vi "Control_Interface_v1.8_cfg.vi"() -> ()   [LabVIEW 2019]
uses:
  Users/zhuen/AppData/Local/CETONI_SDK/lib/labview/labbCAN_Bus_API/labbCAN_Bus_API.lvlib
  Users/zhuen/AppData/Local/CETONI_SDK/lib/labview/labbCAN_Pump_API/labbCAN_Pump_API.lvlib
  Users/zhuen/AppData/Local/CETONI_SDK/lib/labview/labbCAN_Bus_API/TimeUnits.ctl
  Users/zhuen/AppData/Local/CETONI_SDK/lib/labview/labbCAN_Pump_API/VolumeUnits.ctl
  Users/zhuen/AppData/Local/CETONI_SDK/lib/labview/labbCAN_Bus_API/SiUnitPrefix.ctl
panel:
  in  "Tab Control":enum32{"Tracker", "Pump"}(tab)
  in  "Automation":enum16{"OFF", "ON"}(ring)
  in  "Bit Size":enum16{"Auto", "8 bit", "12 bit", "16 bit"}(ring)
  out "Error out Python":errorcluster
  in  "Capture Mode":T1(ring)
  in  "Start Tracker":bool
  out "Tracker  Working":bool
  in  "Browse Capture Path":path
  in  "Capture Path":bool
  in  "File Name":string
  out "Communication Board":string
  in  "Microscopy":enum16{"Fluorescence", "Bright Field"}(ring)
  in  "Tracking Method":enum16{"Contour", "Motion"}(ring)
  in  "Connect":bool
  out "Connected":bool
  out "Config Path":string
  out "Syringe":dbl(slide) caption="Syringe level (ml)" min=0.0 max=10.0 scale=0.0..10.0 scale format="%.1g"
  out "pumping":bool
  in  "SetSyringeLevel":bool
  in  "Generate Flow":bool
  in  "Refill":bool
  in  "Empty":bool
  in  "Stop Dosage":bool
  out "Actual flow rate":dbl caption="Flow rate (ul/min)" format="%#.2g"
  in  "Target Syr Level":dbl caption="Syringe level (ml)" min=0.0 max=10.0 step=1.0 format="%.2g"
  in  "Flow rate":dbl caption="Flow rate (ul/min)" min=-62103.597908503194 max=62103.597908503194 step=1.0 format="%.2g"
  out "Syringe 2":dbl(slide) caption="Syringe level (ml)" min=0.0 max=10.0 scale=0.0..10.0 scale format="%.1g"
  in  "Target Syr Level 2":dbl caption="Syringe level (ml)" min=0.0 max=10.0 step=1.0 format="%.2g"
  in  "Flow rate 2":dbl caption="Flow rate (ul/min)" min=-67160.37941759253 max=67160.37941759253 step=1.0 format="%.2g"
  in  "Stop Dosage 2":bool
  in  "Refill 2":bool
  out "Actual flow rate 2":dbl caption="Flow rate (ul/min)" format="%#.2g"
  out "pumping 2":bool
  in  "Empty 2":bool
  in  "Generate Flow 2":bool
  in  "SetSyringeLevel 2":bool
  out "Syringe 3":dbl(slide) caption="Syringe level (ml)" min=0.0 max=10.0 scale=0.0..10.0 scale format="%.1g"
  in  "Target Syr Level 3":dbl caption="Syringe level (ml)" min=0.0 max=10.0 step=1.0 format="%.2g"
  in  "Flow rate 3":dbl caption="Flow rate (ul/min)" min=-70023.0288619775 max=70023.0288619775 step=1.0 format="%.2g"
  in  "Stop Dosage 3":bool
  in  "Refill 3":bool
  out "Actual flow rate 3":dbl caption="Flow rate (ul/min)" format="%#.2g"
  out "pumping 3":bool
  in  "Empty 3":bool
  in  "Generate Flow 3":bool
  in  "SetSyringeLevel 3":bool
  in  "Total Flow Rate":sgl caption="Total Flow Rate (ul/min)" min=0 max=62103.6 step=1 format="%.2g"
  in  "Stop Dosage All":bool
  in  "Generate Flow All":bool
  out "error out":errorcluster caption="Error pump 1"
  out "error out 2":errorcluster caption="Error pump 2"
  out "error out 3":errorcluster caption="Error pump 3"
  out "Pump handle 3":i64
  out "Pump handle 2":i64
  out "Pump handle":i64
  in  "Interrupt":bool
  in  "Exit":bool
  # "Commands"
  # "Pump"
  # "Target"
  # "Target"
  # "Target"
  # "Actual"
  # "Actual"
  # "Actual"
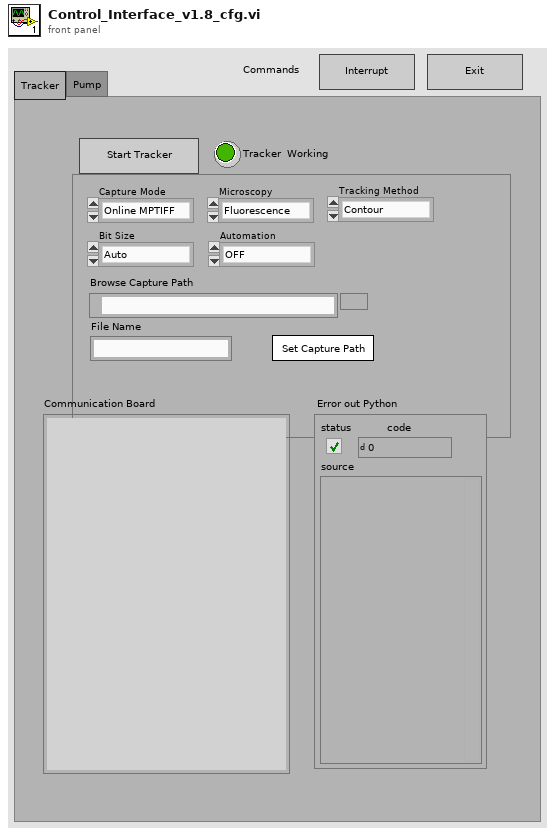
[diagram p1: front panel]
types:
  T1 = enum16{"Online MPTIFF", "Online TIFF", "Offline TIFF"}
  T2 = typedef "labbCAN_Bus_API.lvlib/TimeUnits.ctl" = i32
  T3 = typedef "labbCAN_Pump_API.lvlib/VolumeUnits.ctl" = i32
  T4 = typedef "labbCAN_Bus_API.lvlib/SiUnitPrefix.ctl" = i32
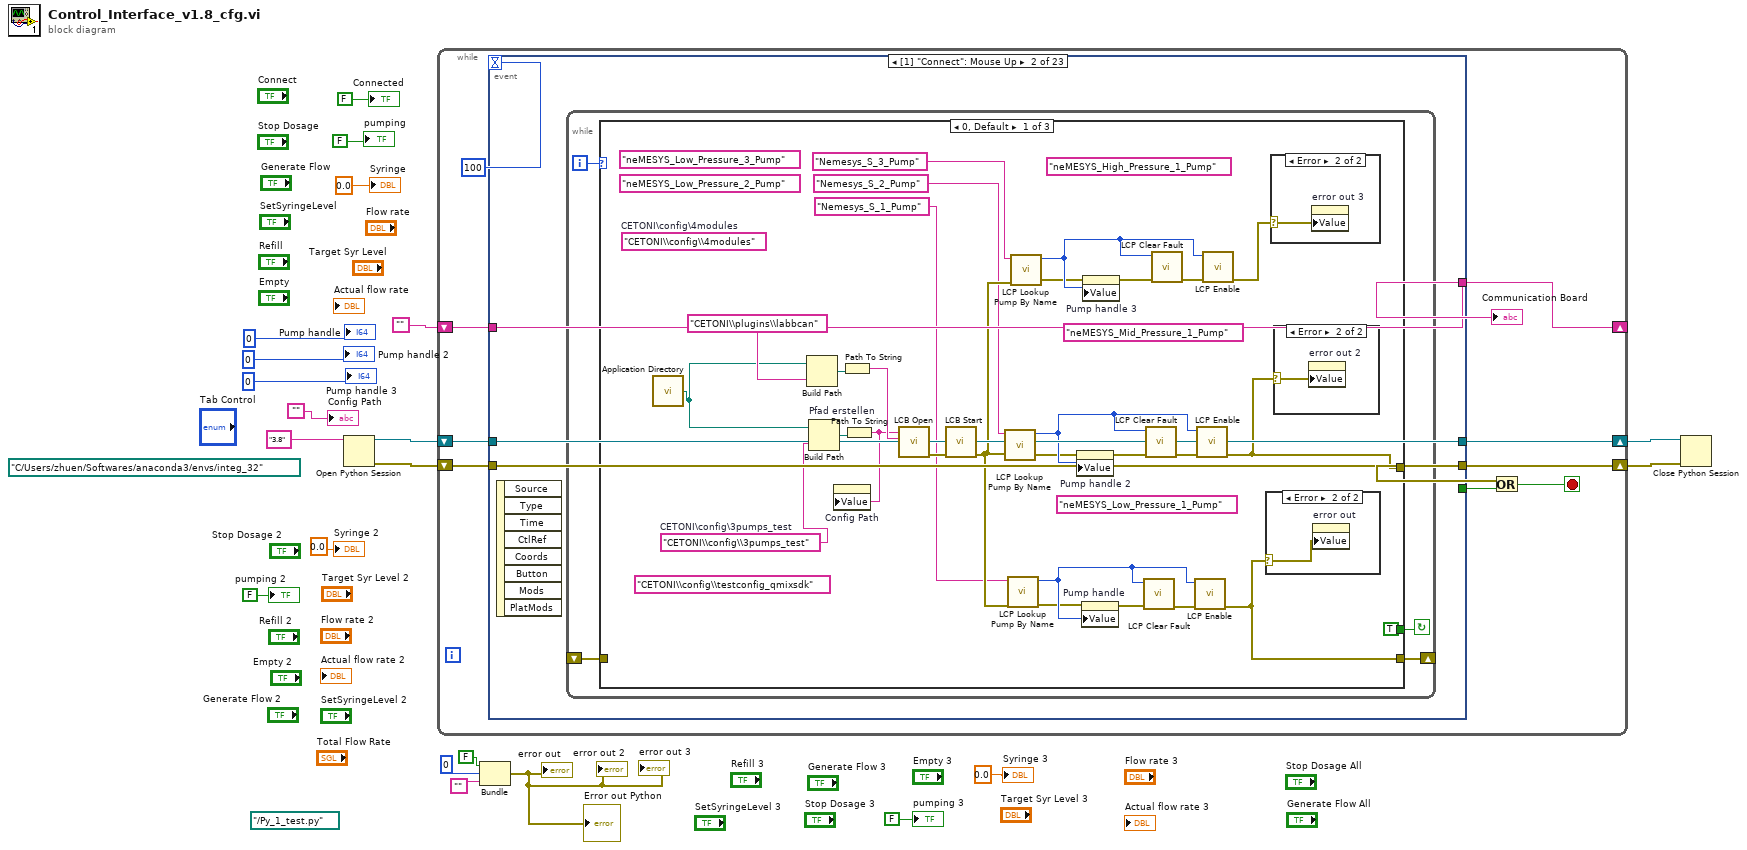
[diagram p0: block diagram]
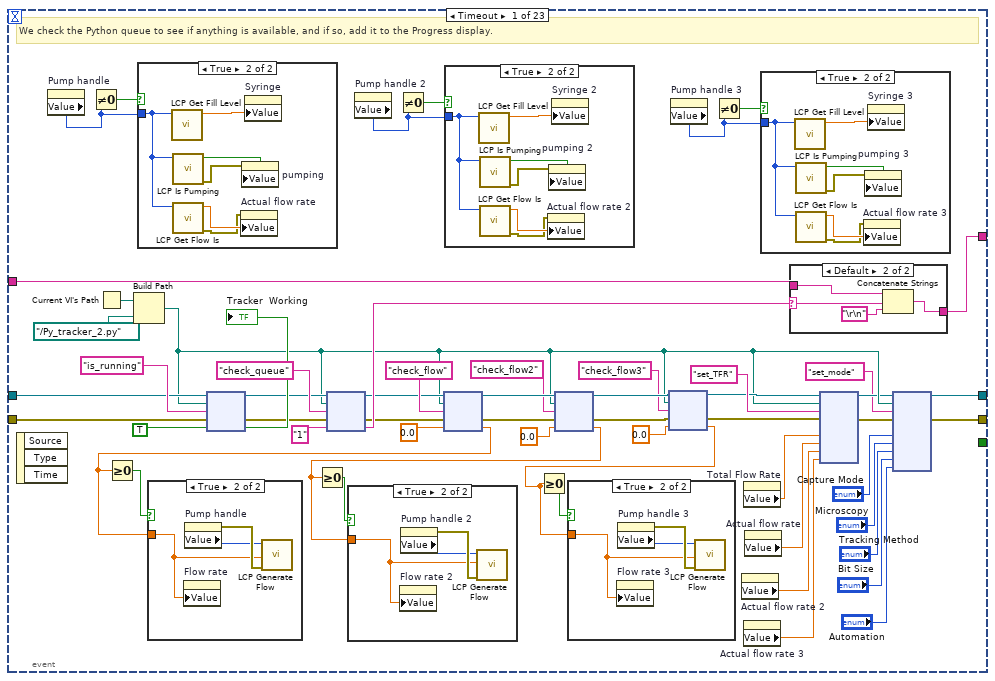
[diagram p2: hidden frame]
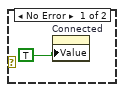
[diagram p10: hidden frame]
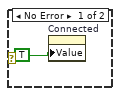
[diagram p11: hidden frame]
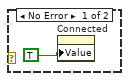
[diagram p12: hidden frame]
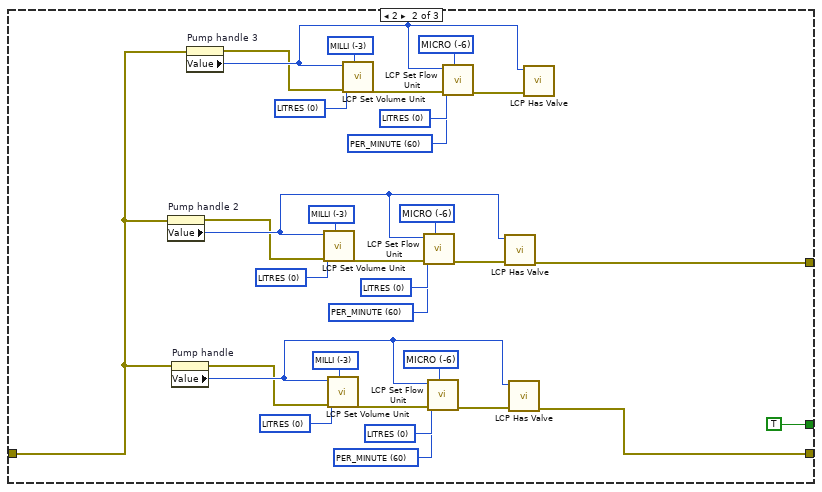
[diagram p13: hidden frame]
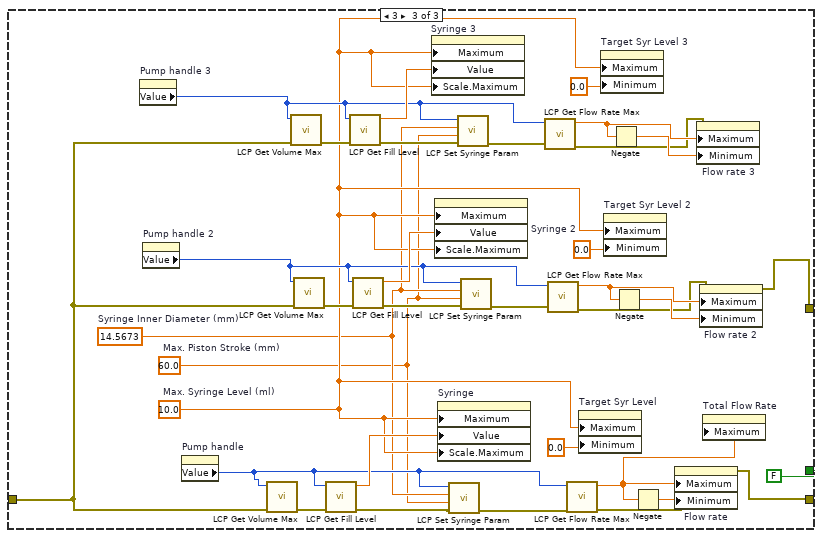
[diagram p14: hidden frame]
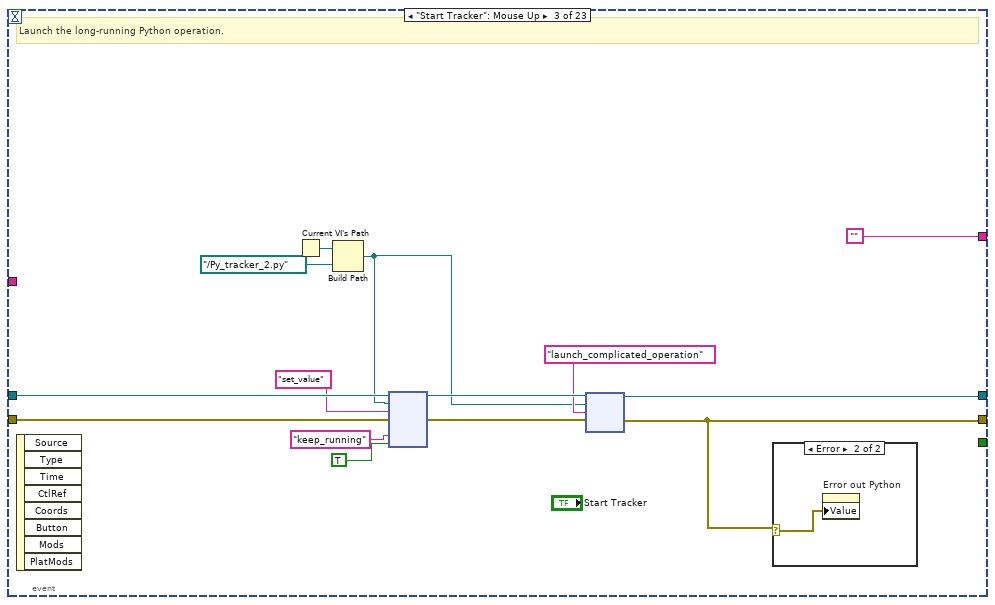
[diagram p15: hidden frame]
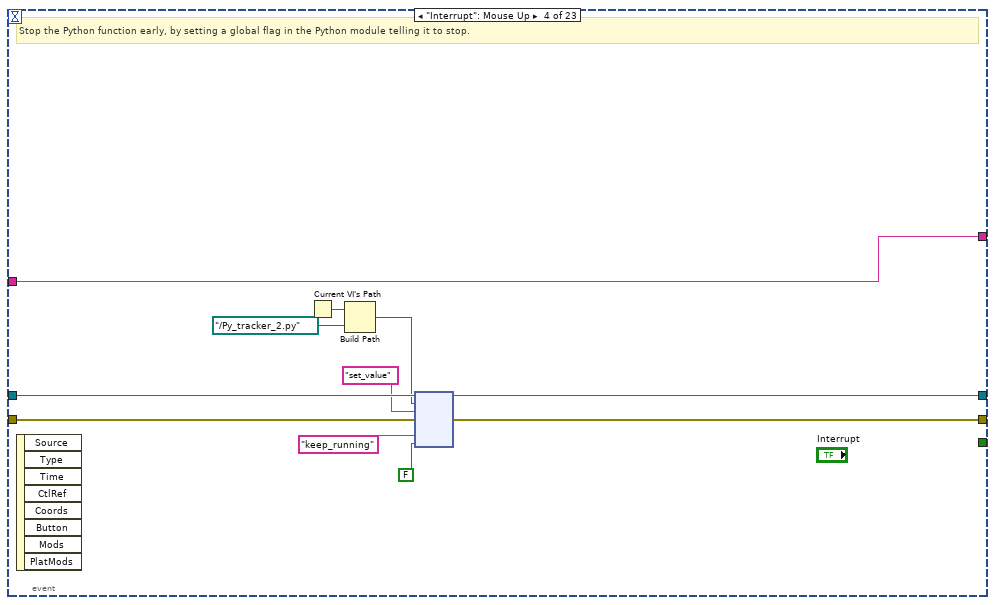
[diagram p17: hidden frame]
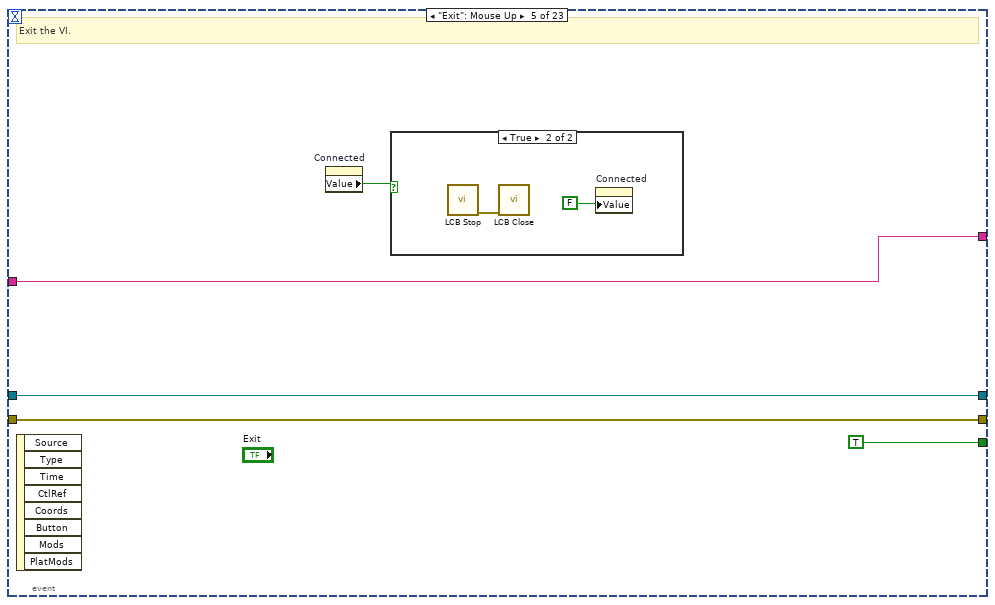
[diagram p18: hidden frame]
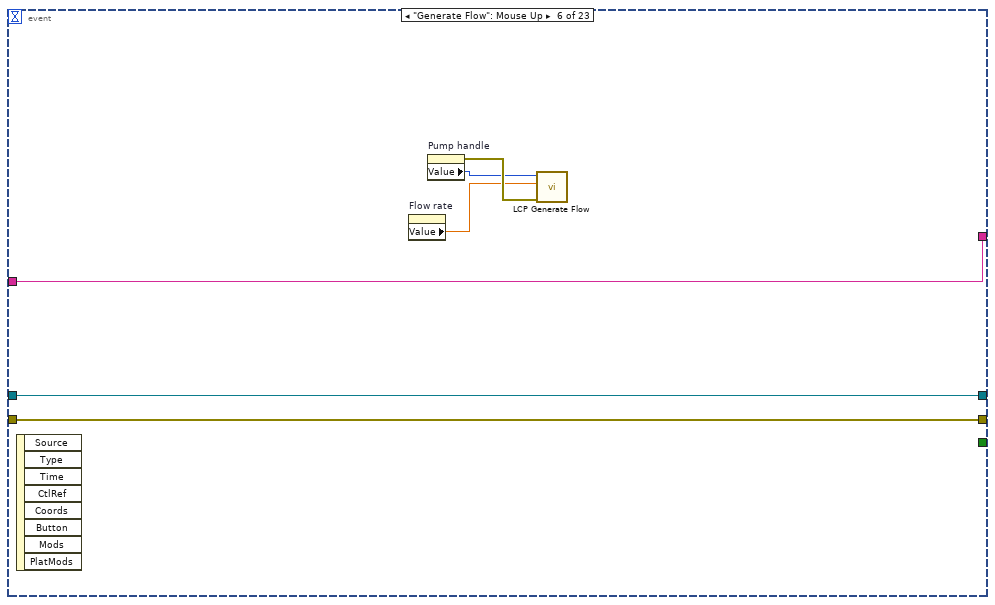
[diagram p20: hidden frame]
diagram:
  (unwired) path "../Py_1_test.py"
  (unwired) path "C:/Users/zhuen/Softwares/anaconda3/envs/integ_32" ("Optional Path to Python.exe")
  n1 = Open Python Session(python version="3.8") -> (session out=w20:refnum<k35>, error out=w19:errorcluster)  [unwired: 2 in]
  n2 = while {
    shift-right: [w26] -> w16
    shift-left: w20 -> [w25]
    shift-right: [w28] -> w17
    shift-left: w19 -> [w29]
    shift-right: [w22] -> _
    shift-left: "" -> [w23]
    stop <- w27 stop-if-true
    n3 = event shown="[1] \"Connect\": Mouse Up" {
      selector: _ -> [_ _ _ _ _ _ _ _ _ _ _ _ _ _ _ _ _ _ _ _ _ _ _]
      dyn-events: _ -> [_ _ _ _ _ _ _ _ _ _ _ _ _ _ _ _ _ _ _ _ _ _ _]
      timeout: 100 -> [_ _ _ _ _ _ _ _ _ _ _ _ _ _ _ _ _ _ _ _ _ _ _]
      tunnel: [_ _ _ _ TRUE _ _ _ _ _ _ _ _ _ _ _ _ _ _ _ _ _ _] -> w30
      tunnel: [w41 w120 w225 w244 w254 w258 w264 w270 w282 w288 w294 w299 w308 w312 w318 w324 w333 w344 w355 w366 w376 w385 w393] -> w28
      tunnel: w29 -> [w82 w120 w232 w245 w254 w258 w264 w270 w282 w288 w294 w299 w308 w312 w318 w324 w333 w344 w355 w366 w376 w385 w396]
      tunnel: [w39 w119 w226 w246 w253 w259 w265 w271 w283 w289 w295 w300 w309 w313 w319 w325 w334 w345 w356 w367 w377 w386 w394] -> w26
      tunnel: w25 -> [w75 w119 w237 w247 w253 w259 w265 w271 w283 w289 w295 w300 w309 w313 w319 w325 w334 w345 w356 w367 w377 w386 w397]
      tunnel: w23 -> [w85 w121 _ w250 w252 w260 w266 w272 w284 w290 w293 w298 w307 w314 w320 w326 w335 w346 w357 w368 w378 w387 w391]
      tunnel: [w86 w121 "" w250 w252 w260 w266 w272 w284 w290 w293 w298 w307 w314 w320 w326 w335 w346 w357 w368 w378 w387 w391] -> w22
      event Timeout {
        # "We check the Python queue to see if anything is available, and if so, add it to the Progress display."
        n4 = event-data() -> ()  [unwired: 1 in, 3 out]
        n5 = property on="Pump handle" class="DigNum (strict)"() -> ("Value"=w73:i64)  [unwired: 2 in, 2 out]
        n6 = Not Equal To 0?(x=w73) -> (x != 0?=w74:bool)
        n7 = Current VI's Path() -> (path=w84:path)
        n8 = Build Path(base path=w84, name or relative path=path "../Py_tracker_2.py") -> (appended path=w43:path)
        n9 = case shown="True" w74 {
          tunnel: w73 -> [_ w110]
          frame False {
          }
          frame True {
            n10 = call "LCP Get Fill Level.vi"("Pump Handle"=w110) -> ("Fill Level"=w111:dbl)  [unwired: 9 in, 1 out]
            n11 = call "LCP Is Pumping.vi"("Pump Handle"=w110) -> ("error out"=w113:errorcluster, "Is pumping"=w112:bool)  [unwired: 9 in]
            n12 = call "LCP Get Flow Is.vi"("Pump Handle"=w110) -> ("error out"=w108:errorcluster, "Actual Flow Rate"=w109:dbl)  [unwired: 9 in]
            n13 = property on="Actual flow rate" class="DigNum (strict)"(error in=w108, "Value"=w109) -> ()  [unwired: 1 in, 2 out]
            n14 = property on="pumping" class="Bool (strict)"(error in=w113, "Value"=w112) -> ()  [unwired: 1 in, 2 out]
            n15 = property on="Syringe" class="Slide (strict)"("Value"=w111) -> ()  [unwired: 2 in, 2 out]
          }
        }
        n16 = node(w75, w43, "is_running" ("Function or Method Name"), w82, TRUE) -> (w72:refnum<k35>, w71:errorcluster, →"Tracker  Working":bool)  [unwired: 2 out]
        n17 = node(w72, w43, "check_queue" ("Function or Method Name"), w71, "1") -> (w69:refnum<k35>, w68:errorcluster, w77:string)  [unwired: 2 out]
        n18 = property on="Pump handle 2" class="DigNum (strict)"() -> ("Value"=w59:i64)  [unwired: 2 in, 2 out]
        n19 = Not Equal To 0?(x=w59) -> (x != 0?=w60:bool)
        n20 = node(w69, w43, "check_flow" ("Function or Method Name"), w68, 0.0) -> (w65:refnum<k35>, w64:errorcluster, w66:dbl)  [unwired: 2 out]
        n21 = Greater Or Equal To 0?(x=w66) -> (x >= 0?=w67:bool)
        n22 = case shown="True" w67 {
          tunnel: w66 -> [_ w105]
          frame False {
          }
          frame True {
            n23 = property on="Flow rate" class="DigNum (strict)"("Value"=w105) -> ()  [unwired: 2 in, 2 out]
            n24 = property on="Pump handle" class="DigNum (strict)"() -> (error out=w107:errorcluster, "Value"=w106:i64)  [unwired: 2 in, 1 out]
            n25 = call "LCP Generate Flow.vi"("error in (no error)"=w107, "Flow Rate"=w105, "Pump Handle"=w106) -> ()  [unwired: 8 in, 1 out]
          }
        }
        n26 = case shown="True" w60 {
          tunnel: w59 -> [_ w98]
          frame False {
          }
          frame True {
            n27 = call "LCP Get Fill Level.vi"("Pump Handle"=w98) -> ("Fill Level"=w99:dbl)  [unwired: 9 in, 1 out]
            n28 = call "LCP Is Pumping.vi"("Pump Handle"=w98) -> ("error out"=w101:errorcluster, "Is pumping"=w100:bool)  [unwired: 9 in]
            n29 = call "LCP Get Flow Is.vi"("Pump Handle"=w98) -> ("error out"=w96:errorcluster, "Actual Flow Rate"=w97:dbl)  [unwired: 9 in]
            n30 = property on="Actual flow rate 2" class="DigNum (strict)"(error in=w96, "Value"=w97) -> ()  [unwired: 1 in, 2 out]
            n31 = property on="pumping 2" class="Bool (strict)"(error in=w101, "Value"=w100) -> ()  [unwired: 1 in, 2 out]
            n32 = property on="Syringe 2" class="Slide (strict)"("Value"=w99) -> ()  [unwired: 2 in, 2 out]
          }
        }
        n33 = node(w65, w43, "check_flow2" ("Function or Method Name"), w64, 0.0) -> (w52:refnum<k35>, w50:errorcluster, w61:dbl)  [unwired: 2 out]
        n34 = Greater Or Equal To 0?(x=w61) -> (x >= 0?=w62:bool)
        n35 = case shown="True" w62 {
          tunnel: w61 -> [_ w102]
          frame False {
          }
          frame True {
            n36 = property on="Flow rate 2" class="DigNum (strict)"("Value"=w102) -> ()  [unwired: 2 in, 2 out]
            n37 = property on="Pump handle 2" class="DigNum (strict)"() -> (error out=w104:errorcluster, "Value"=w103:i64)  [unwired: 2 in, 1 out]
            n38 = call "LCP Generate Flow.vi"("error in (no error)"=w104, "Flow Rate"=w102, "Pump Handle"=w103) -> ()  [unwired: 8 in, 1 out]
          }
        }
        n39 = node(w52, w43, "check_flow3" ("Function or Method Name"), w50, 0.0) -> (w51:refnum<k35>, w49:errorcluster, w45:dbl)  [unwired: 2 out]
        n40 = Greater Or Equal To 0?(x=w45) -> (x >= 0?=w46:bool)
        n41 = case shown="True" w46 {
          tunnel: w45 -> [_ w87]
          frame False {
          }
          frame True {
            n42 = property on="Flow rate 3" class="DigNum (strict)"("Value"=w87) -> ()  [unwired: 2 in, 2 out]
            n43 = property on="Pump handle 3" class="DigNum (strict)"() -> (error out=w89:errorcluster, "Value"=w88:i64)  [unwired: 2 in, 1 out]
            n44 = call "LCP Generate Flow.vi"("error in (no error)"=w89, "Flow Rate"=w87, "Pump Handle"=w88) -> ()  [unwired: 8 in, 1 out]
          }
        }
        n45 = property on="Pump handle 3" class="DigNum (strict)"() -> ("Value"=w53:i64)  [unwired: 2 in, 2 out]
        n46 = Not Equal To 0?(x=w53) -> (x != 0?=w54:bool)
        n47 = property on="Actual flow rate 2" class="DigNum (strict)"() -> ("Value"=w33:dbl)  [unwired: 2 in, 2 out]
        n48 = property on="Total Flow Rate" class="DigNum (strict)"() -> ("Value"=w55:sgl)  [unwired: 2 in, 2 out]
        n49 = property on="Actual flow rate 3" class="DigNum (strict)"() -> ("Value"=w32:dbl)  [unwired: 2 in, 2 out]
        n50 = property on="Actual flow rate" class="DigNum (strict)"() -> ("Value"=w34:dbl)  [unwired: 2 in, 2 out]
        n51 = case shown="True" w54 {
          tunnel: w53 -> [_ w92]
          frame False {
          }
          frame True {
            n52 = call "LCP Get Fill Level.vi"("Pump Handle"=w92) -> ("Fill Level"=w93:dbl)  [unwired: 9 in, 1 out]
            n53 = call "LCP Is Pumping.vi"("Pump Handle"=w92) -> ("error out"=w95:errorcluster, "Is pumping"=w94:bool)  [unwired: 9 in]
            n54 = call "LCP Get Flow Is.vi"("Pump Handle"=w92) -> ("error out"=w90:errorcluster, "Actual Flow Rate"=w91:dbl)  [unwired: 9 in]
            n55 = property on="Actual flow rate 3" class="DigNum (strict)"(error in=w90, "Value"=w91) -> ()  [unwired: 1 in, 2 out]
            n56 = property on="pumping 3" class="Bool (strict)"(error in=w95, "Value"=w94) -> ()  [unwired: 1 in, 2 out]
            n57 = property on="Syringe 3" class="Slide (strict)"("Value"=w93) -> ()  [unwired: 2 in, 2 out]
          }
        }
        n58 = case shown="Default" w77 {
          selector: w77 -> [_ w115]
          tunnel: [w114 w118] -> w86
          tunnel: w85 -> [w114 w116]
          frame "" {
          }
          frame Default {
            n59 = Concatenate Strings(w116, w115, "\r\n") -> (w118:string)
          }
        }
        n60 = node(w51, w43, "set_TFR" ("Function or Method Name"), w49, w55, w34, w33, w32) -> (w40:refnum<k35>, w42:errorcluster)  [unwired: 6 in, 2 out]
        n61 = node(w40, w43, "set_mode" ("Function or Method Name"), w42, "Capture Mode", "Microscopy", "Tracking Method", "Bit Size", "Automation") -> (w39:refnum<k35>, w41:errorcluster)  [unwired: 7 in, 2 out]
      }
      event "Connect": Mouse Up {
        n62 = event-data() -> ()  [unwired: 1 in, 8 out]
        n63 = while {
          shift-right: [w123] -> _
          shift-left: _ -> [w122]
          i -> [w125]
          stop <- w124 continue-if-true
          n64 = case shown="0, Default" w125 {
            tunnel: [TRUE TRUE FALSE] -> w124
            tunnel: [w145 w171 w220] -> w123
            tunnel: w122 -> [_ w160 w195]
            tunnel: [w141 w170 w192] -> _
            frame 0, Default {
              (unwired) "CETONI\\config\\4modules"  # CETONI\config\4modules
              (unwired) "neMESYS_Low_Pressure_2_Pump"
              (unwired) "neMESYS_Low_Pressure_3_Pump"
              (unwired) "neMESYS_Low_Pressure_1_Pump" ("pAxisName")
              (unwired) "neMESYS_Mid_Pressure_1_Pump" ("pAxisName")
              (unwired) "neMESYS_High_Pressure_1_Pump" ("pAxisName")
              w126 = "CETONI\\config\\3pumps_test"  # CETONI\config\3pumps_test
              (unwired) "CETONI\\config\\testconfig_qmixsdk" ("Name oder relativer Pfad")
              n65 = call <vilib>:"Application Directory.vi"() -> ("Application Directory"=w146:path)
              n66 = Build Path(base path=w146, name or relative path="CETONI\\plugins\\labbcan" ("Name oder relativer Pfad")) -> (appended path=w153:path)
              n67 = Build Path "Pfad erstellen"(base path=w146, name or relative path=w126) -> (appended path=w152:path)
              n68 = Path To String(path=w153) -> (string=w140:string)
              n69 = Path To String(path=w152) -> (string=w139:string)
              n70 = property on="Config Path" class="Str"("Value"=w139) -> ()  [unwired: 2 in, 2 out]
              n71 = call "LCB Open.vi"("PluginSearchPath"=w140, "Device Configuration Path"=w139) -> ("error out"=w136:errorcluster)  [unwired: 9 in]
              n72 = call "LCB Start.vi"("error in (no error)"=w136) -> ("error out"=w131:errorcluster)  [unwired: 10 in]
              n73 = call "LCP Lookup Pump By Name.vi"("error in (no error)"=w131, "Pump Name"="Nemesys_S_2_Pump" ("pAxisName")) -> ("error out"=w142:errorcluster, "Pump handle"=w143:i64)  [unwired: 8 in]
              n74 = call "LCP Lookup Pump By Name.vi"("error in (no error)"=w131, "Pump Name"="Nemesys_S_1_Pump" ("pAxisName")) -> ("error out"=w147:errorcluster, "Pump handle"=w148:i64)  [unwired: 8 in]
              n75 = call "LCP Lookup Pump By Name.vi"("error in (no error)"=w131, "Pump Name"="Nemesys_S_3_Pump" ("pAxisName")) -> ("error out"=w133:errorcluster, "Pump handle"=w134:i64)  [unwired: 8 in]
              n76 = property on="Pump handle 2" class="DigNum (strict)"(error in=w142, "Value"=w143) -> (error out=w138:errorcluster)  [unwired: 1 in, 1 out]
              n77 = property on="Pump handle" class="DigNum (strict)"(error in=w147, "Value"=w148) -> (error out=w137:errorcluster)  [unwired: 1 in, 1 out]
              n78 = property on="Pump handle 3" class="DigNum (strict)"(error in=w133, "Value"=w134) -> (error out=w132:errorcluster)  [unwired: 1 in, 1 out]
              n79 = call "LCP Clear Fault.vi"("error in (no error)"=w137, "Pump Handle"=w148) -> ("error out"=w151:errorcluster)  [unwired: 9 in]
              n80 = call "LCP Clear Fault.vi"("error in (no error)"=w138, "Pump Handle"=w143) -> ("error out"=w144:errorcluster)  [unwired: 9 in]
              n81 = call "LCP Clear Fault.vi"("error in (no error)"=w132, "Pump Handle"=w134) -> ("error out"=w135:errorcluster)  [unwired: 9 in]
              n82 = call "LCP Enable.vi"("error in (no error)"=w151, "Pump Handle"=w148) -> ("error out"=w145:errorcluster)  [unwired: 9 in]
              n83 = call "LCP Enable.vi"("error in (no error)"=w144, "Pump Handle"=w143) -> ("error out"=w141:errorcluster)  [unwired: 9 in]
              n84 = call "LCP Enable.vi"("error in (no error)"=w135, "Pump Handle"=w134) -> ("error out"=w130:errorcluster)  [unwired: 9 in]
              n85 = case shown="Error" w145 {
                selector: w145 -> [_ w159]
                frame No Error {
                  n86 = property on="Connected" class="Bool (strict)"("Value"=TRUE ("Connected")) -> ()  [unwired: 2 in, 2 out]
                }
                frame Error {
                  n87 = property on="error out" class="Clust (strict)"("Value"=w159) -> ()  [unwired: 2 in, 2 out]
                }
              }
              n88 = case shown="Error" w130 {
                selector: w130 -> [_ w155]
                frame No Error {
                  n89 = property on="Connected" class="Bool (strict)"("Value"=TRUE ("Connected")) -> ()  [unwired: 2 in, 2 out]
                }
                frame Error {
                  n90 = property on="error out 3" class="Clust (strict)"("Value"=w155) -> ()  [unwired: 2 in, 2 out]
                }
              }
              n91 = case shown="Error" w141 {
                selector: w141 -> [_ w157]
                frame No Error {
                  n92 = property on="Connected" class="Bool (strict)"("Value"=TRUE ("Connected")) -> ()  [unwired: 2 in, 2 out]
                }
                frame Error {
                  n93 = property on="error out 2" class="Clust (strict)"("Value"=w157) -> ()  [unwired: 2 in, 2 out]
                }
              }
            }
            frame 2 {
              w164 = T2 60 items=["PER_SECOND"=1, "PER_MINUTE"=60, "PER_HOUR"=3600] ("TimeUnit")
              w165 = T3 0 items=["LITRES"] ("VolumeUnit")
              w166 = T3 0 items=["LITRES"] ("Volume Unit")
              w167 = T4 -6 items=["UNIT"=0, "DECI"=-1, "CENTI"=-2, "MILLI"=-3, "MICRO"=-6] ("Prefix")
              w169 = T4 -3 items=["UNIT"=0, "DECI"=-1, "CENTI"=-2, "MILLI"=-3, "MICRO"=-6] ("Prefix")
              w175 = T2 60 items=["PER_SECOND"=1, "PER_MINUTE"=60, "PER_HOUR"=3600] ("TimeUnit")
              w176 = T3 0 items=["LITRES"] ("VolumeUnit")
              w177 = T3 0 items=["LITRES"] ("Volume Unit")
              w178 = T4 -6 items=["UNIT"=0, "DECI"=-1, "CENTI"=-2, "MILLI"=-3, "MICRO"=-6] ("Prefix")
              w180 = T4 -3 items=["UNIT"=0, "DECI"=-1, "CENTI"=-2, "MILLI"=-3, "MICRO"=-6] ("Prefix")
              w184 = T2 60 items=["PER_SECOND"=1, "PER_MINUTE"=60, "PER_HOUR"=3600] ("TimeUnit")
              w185 = T3 0 items=["LITRES"] ("VolumeUnit")
              w186 = T3 0 items=["LITRES"] ("Volume Unit")
              w187 = T4 -6 items=["UNIT"=0, "DECI"=-1, "CENTI"=-2, "MILLI"=-3, "MICRO"=-6] ("Prefix")
              w189 = T4 -3 items=["UNIT"=0, "DECI"=-1, "CENTI"=-2, "MILLI"=-3, "MICRO"=-6] ("Prefix")
              n94 = property on="Pump handle 2" class="DigNum (strict)"(error in=w160) -> (error out=w172:errorcluster, "Value"=w173:i64)  [unwired: 1 in, 1 out]
              n95 = property on="Pump handle" class="DigNum (strict)"(error in=w160) -> (error out=w181:errorcluster, "Value"=w182:i64)  [unwired: 1 in, 1 out]
              n96 = property on="Pump handle 3" class="DigNum (strict)"(error in=w160) -> (error out=w161:errorcluster, "Value"=w162:i64)  [unwired: 1 in, 1 out]
              n97 = call "LCP Set Volume Unit.vi"("Prefix"=w180, "error in (no error)"=w172, "Volume Unit"=w177, "Pump Handle"=w173) -> ("error out"=w179:errorcluster)  [unwired: 7 in]
              n98 = call "LCP Set Volume Unit.vi"("Prefix"=w189, "error in (no error)"=w181, "Volume Unit"=w186, "Pump Handle"=w182) -> ("error out"=w188:errorcluster)  [unwired: 7 in]
              n99 = call "LCP Set Volume Unit.vi"("Prefix"=w169, "error in (no error)"=w161, "Volume Unit"=w166, "Pump Handle"=w162) -> ("error out"=w168:errorcluster)  [unwired: 7 in]
              n100 = call "LCP Set Flow Unit.vi"("Prefix"=w178, "error in (no error)"=w179, "TimeUnit"=w175, "VolumeUnit"=w176, "Pump Handle"=w173) -> ("error out"=w174:errorcluster)  [unwired: 6 in]
              n101 = call "LCP Set Flow Unit.vi"("Prefix"=w187, "error in (no error)"=w188, "TimeUnit"=w184, "VolumeUnit"=w185, "Pump Handle"=w182) -> ("error out"=w183:errorcluster)  [unwired: 6 in]
              n102 = call "LCP Set Flow Unit.vi"("Prefix"=w167, "error in (no error)"=w168, "TimeUnit"=w164, "VolumeUnit"=w165, "Pump Handle"=w162) -> ("error out"=w163:errorcluster)  [unwired: 6 in]
              n103 = call "LCP Has Valve.vi"("error in (no error)"=w174, "Pump Handle"=w173) -> ("error out"=w170:errorcluster)  [unwired: 8 in, 1 out]
              n104 = call "LCP Has Valve.vi"("error in (no error)"=w183, "Pump Handle"=w182) -> ("error out"=w171:errorcluster)  [unwired: 8 in, 1 out]
              n105 = call "LCP Has Valve.vi"("error in (no error)"=w163, "Pump Handle"=w162) -> ()  [unwired: 8 in, 2 out]
            }
            frame 3 {
              w191 = 60.0  # Max. Piston Stroke (mm)
              w193 = 14.5673  # Syringe Inner Diameter (mm)
              w194 = 10.0  # Max. Syringe Level (ml)
              n106 = property on="Pump handle 3" class="DigNum (strict)"() -> ("Value"=w198:i64)  [unwired: 2 in, 2 out]
              n107 = property on="Pump handle 2" class="DigNum (strict)"() -> ("Value"=w207:i64)  [unwired: 2 in, 2 out]
              n108 = property on="Pump handle" class="DigNum (strict)"() -> ("Value"=w208:i64)  [unwired: 2 in, 2 out]
              n109 = call "LCP Get Volume Max.vi"("error in (no error)"=w195, "Pump Handle"=w208) -> ("error out"=w223:errorcluster)  [unwired: 8 in, 1 out]
              n110 = call "LCP Get Volume Max.vi"("error in (no error)"=w195, "Pump Handle"=w198) -> ("error out"=w204:errorcluster)  [unwired: 8 in, 1 out]
              n111 = call "LCP Get Volume Max.vi"("error in (no error)"=w195, "Pump Handle"=w207) -> ("error out"=w217:errorcluster)  [unwired: 8 in, 1 out]
              n112 = call "LCP Get Fill Level.vi"("error in (no error)"=w223, "Pump Handle"=w208) -> ("error out"=w210:errorcluster, "Fill Level"=w222:dbl)  [unwired: 8 in]
              n113 = call "LCP Get Fill Level.vi"("error in (no error)"=w204, "Pump Handle"=w198) -> ("error out"=w197:errorcluster, "Fill Level"=w202:dbl)  [unwired: 8 in]
              n114 = call "LCP Get Fill Level.vi"("error in (no error)"=w217, "Pump Handle"=w207) -> ("error out"=w206:errorcluster, "Fill Level"=w215:dbl)  [unwired: 8 in]
              n115 = property on="Syringe 3" class="Slide (strict)"("Maximum"=w194, "Value"=w202, "Scale.Maximum"=w194) -> ()  [unwired: 2 in, 2 out]
              n116 = property on="Syringe 2" class="Slide (strict)"("Maximum"=w194, "Value"=w215, "Scale.Maximum"=w194) -> ()  [unwired: 2 in, 2 out]
              n117 = property on="Syringe" class="Slide (strict)"("Maximum"=w194, "Value"=w222, "Scale.Maximum"=w194) -> ()  [unwired: 2 in, 2 out]
              n118 = call "LCP Set Syringe Param.vi"("error in (no error)"=w210, "Maximum Piston Stroke (mm)"=w191, "Inner Diameter (mm)"=w193, "Pump Handle"=w208) -> ("error out"=w209:errorcluster)  [unwired: 7 in]
              n119 = call "LCP Set Syringe Param.vi"("error in (no error)"=w197, "Maximum Piston Stroke (mm)"=w191, "Inner Diameter (mm)"=w193, "Pump Handle"=w198) -> ("error out"=w196:errorcluster)  [unwired: 7 in]
              n120 = call "LCP Set Syringe Param.vi"("error in (no error)"=w206, "Maximum Piston Stroke (mm)"=w191, "Inner Diameter (mm)"=w193, "Pump Handle"=w207) -> ("error out"=w205:errorcluster)  [unwired: 7 in]
              n121 = call "LCP Get Flow Rate Max.vi"("error in (no error)"=w196, "Pump Handle"=w198) -> ("error out"=w199:errorcluster, "Maximum Flow Rate"=w201:dbl)  [unwired: 8 in]
              n122 = call "LCP Get Flow Rate Max.vi"("error in (no error)"=w205, "Pump Handle"=w207) -> ("error out"=w212:errorcluster, "Maximum Flow Rate"=w214:dbl)  [unwired: 8 in]
              n123 = call "LCP Get Flow Rate Max.vi"("error in (no error)"=w209, "Pump Handle"=w208) -> ("error out"=w221:errorcluster, "Maximum Flow Rate"=w211:dbl)  [unwired: 8 in]
              n124 = property on="Target Syr Level" class="DigNum (strict)"("Maximum"=w194, "Minimum"=0.0 ("Wertebereich:Minimum")) -> ()  [unwired: 2 in, 2 out]
              n125 = property on="Target Syr Level 3" class="DigNum (strict)"("Maximum"=w194, "Minimum"=0.0 ("Wertebereich:Minimum")) -> ()  [unwired: 2 in, 2 out]
              n126 = property on="Target Syr Level 2" class="DigNum (strict)"("Maximum"=w194, "Minimum"=0.0 ("Wertebereich:Minimum")) -> ()  [unwired: 2 in, 2 out]
              n127 = Negate(x=w201) -> (-x=w200:dbl)
              n128 = Negate(x=w214) -> (-x=w213:dbl)
              n129 = Negate(x=w211) -> (-x=w219:dbl)
              n130 = property on="Flow rate" class="DigNum (strict)"(error in=w221, "Maximum"=w211, "Minimum"=w219) -> (error out=w220:errorcluster)  [unwired: 1 in, 1 out]
              n131 = property on="Flow rate 3" class="DigNum (strict)"(error in=w199, "Maximum"=w201, "Minimum"=w200) -> ()  [unwired: 1 in, 2 out]
              n132 = property on="Flow rate 2" class="DigNum (strict)"(error in=w212, "Maximum"=w214, "Minimum"=w213) -> (error out=w192:errorcluster)  [unwired: 1 in, 1 out]
              n133 = property on="Total Flow Rate" class="DigNum (strict)"("Maximum"=w211) -> ()  [unwired: 2 in, 2 out]
            }
          }
        }
      }
      event "Start Tracker": Mouse Up {
        # "Launch the long-running Python operation."
        n134 = event-data() -> ()  [unwired: 1 in, 8 out]
        n135 = Current VI's Path() -> (path=w235:path)
        n136 = Build Path(base path=w235, name or relative path=path "../Py_tracker_2.py") -> (appended path=w227:path)
        n137 = node(w237, w227, "set_value", w232, "keep_running" ("Object Name"), TRUE) -> (w230:refnum<k35>, w229:errorcluster)  [unwired: 4 in, 2 out]
        n138 = node(w230, w227, "launch_complicated_operation" ("Function or Method Name"), w229) -> (w226:refnum<k35>, w225:errorcluster)  [unwired: 2 in, 2 out]
        n139 = case shown="Error" w225 {
          selector: w225 -> [_ w239]
          frame No Error {
          }
          frame Error {
            n140 = property on="Error out Python" class="Clust (strict)"("Value"=w239) -> ()  [unwired: 2 in, 2 out]
          }
        }
      }
      event "Interrupt": Mouse Up {
        # "Stop the Python function early, by setting a global flag in the Python module telling it to stop."
        n141 = event-data() -> ()  [unwired: 1 in, 8 out]
        n142 = Current VI's Path() -> (path=w249:path)
        n143 = Build Path(base path=w249, name or relative path=path "../Py_tracker_2.py") -> (appended path=w242:path)
        n144 = node(w247, w242, "set_value", w245, "keep_running" ("Object Name"), FALSE) -> (w246:refnum<k35>, w244:errorcluster)  [unwired: 4 in, 2 out]
      }
      event "Exit": Mouse Up {
        # "Exit the VI."
        n145 = event-data() -> ()  [unwired: 1 in, 8 out]
        n146 = property on="Connected" class="Bool (strict)"() -> ("Value"=w251:bool)  [unwired: 2 in, 2 out]
        n147 = case shown="True" w251 {
          frame False {
          }
          frame True {
            n148 = call "LCB Stop.vi"() -> ("error out"=w257:errorcluster)  [unwired: 11 in]
            n149 = call "LCB Close.vi"("error in (no error)"=w257) -> ()  [unwired: 10 in, 1 out]
            n150 = property on="Connected" class="Bool (strict)"("Value"=FALSE) -> ()  [unwired: 2 in, 2 out]
          }
        }
      }
      event "Generate Flow": Mouse Up {
        n151 = event-data() -> ()  [unwired: 1 in, 8 out]
        n152 = property on="Flow rate" class="DigNum (strict)"() -> ("Value"=w262:dbl)  [unwired: 2 in, 2 out]
        n153 = property on="Pump handle" class="DigNum (strict)"() -> (error out=w263:errorcluster, "Value"=w261:i64)  [unwired: 2 in, 1 out]
        n154 = call "LCP Generate Flow.vi"("error in (no error)"=w263, "Flow Rate"=w262, "Pump Handle"=w261) -> ()  [unwired: 8 in, 1 out]
      }
      event "Generate Flow 2": Mouse Up {
        n155 = event-data() -> ()  [unwired: 1 in, 8 out]
        n156 = property on="Flow rate 2" class="DigNum (strict)"() -> ("Value"=w268:dbl)  [unwired: 2 in, 2 out]
        n157 = property on="Pump handle 2" class="DigNum (strict)"() -> (error out=w269:errorcluster, "Value"=w267:i64)  [unwired: 2 in, 1 out]
        n158 = call "LCP Generate Flow.vi"("error in (no error)"=w269, "Flow Rate"=w268, "Pump Handle"=w267) -> ()  [unwired: 8 in, 1 out]
      }
      event "Generate Flow 3": Mouse Up {
        n159 = event-data() -> ()  [unwired: 1 in, 8 out]
        n160 = property on="Flow rate 3" class="DigNum (strict)"() -> ("Value"=w274:dbl)  [unwired: 2 in, 2 out]
        n161 = property on="Pump handle 3" class="DigNum (strict)"() -> (error out=w275:errorcluster, "Value"=w273:i64)  [unwired: 2 in, 1 out]
        n162 = call "LCP Generate Flow.vi"("error in (no error)"=w275, "Flow Rate"=w274, "Pump Handle"=w273) -> ()  [unwired: 8 in, 1 out]
      }
      event "Generate Flow All": Mouse Up {
        n163 = event-data() -> ()  [unwired: 1 in, 8 out]
        n164 = property on="Flow rate" class="DigNum (strict)"() -> ("Value"=w277:dbl)  [unwired: 2 in, 2 out]
        n165 = property on="Pump handle" class="DigNum (strict)"() -> (error out=w281:errorcluster, "Value"=w280:i64)  [unwired: 2 in, 1 out]
        n166 = call "LCP Generate Flow.vi"("error in (no error)"=w281, "Flow Rate"=w277, "Pump Handle"=w280) -> ()  [unwired: 8 in, 1 out]
        n167 = property on="Flow rate 2" class="DigNum (strict)"() -> ("Value"=w276:dbl)  [unwired: 2 in, 2 out]
        n168 = property on="Pump handle 2" class="DigNum (strict)"() -> (error out=w279:errorcluster, "Value"=w278:i64)  [unwired: 2 in, 1 out]
        n169 = call "LCP Generate Flow.vi"("error in (no error)"=w279, "Flow Rate"=w276, "Pump Handle"=w278) -> ()  [unwired: 8 in, 1 out]
        n170 = property on="Flow rate 3" class="DigNum (strict)"() -> ("Value"=w286:dbl)  [unwired: 2 in, 2 out]
        n171 = property on="Pump handle 3" class="DigNum (strict)"() -> (error out=w287:errorcluster, "Value"=w285:i64)  [unwired: 2 in, 1 out]
        n172 = call "LCP Generate Flow.vi"("error in (no error)"=w287, "Flow Rate"=w286, "Pump Handle"=w285) -> ()  [unwired: 8 in, 1 out]
      }
      event "Stop Dosage": Mouse Up {
        n173 = event-data() -> ()  [unwired: 1 in, 8 out]
        n174 = property on="Pump handle" class="DigNum (strict)"() -> (error out=w292:errorcluster, "Value"=w291:i64)  [unwired: 2 in, 1 out]
        n175 = call "LCP Stop Pumping.vi"("error in (no error)"=w292, "Pump Handle"=w291) -> ()  [unwired: 9 in, 1 out]
      }
      event "Stop Dosage 2": Mouse Up {
        n176 = event-data() -> ()  [unwired: 1 in, 8 out]
        n177 = property on="Pump handle 2" class="DigNum (strict)"() -> (error out=w297:errorcluster, "Value"=w296:i64)  [unwired: 2 in, 1 out]
        n178 = call "LCP Stop Pumping.vi"("error in (no error)"=w297, "Pump Handle"=w296) -> ()  [unwired: 9 in, 1 out]
      }
      event "Stop Dosage 3": Mouse Up {
        n179 = event-data() -> ()  [unwired: 1 in, 8 out]
        n180 = property on="Pump handle 3" class="DigNum (strict)"() -> (error out=w302:errorcluster, "Value"=w301:i64)  [unwired: 2 in, 1 out]
        n181 = call "LCP Stop Pumping.vi"("error in (no error)"=w302, "Pump Handle"=w301) -> ()  [unwired: 9 in, 1 out]
      }
      event "Stop Dosage All": Mouse Up {
        n182 = event-data() -> ()  [unwired: 1 in, 8 out]
        n183 = property on="Pump handle" class="DigNum (strict)"() -> (error out=w306:errorcluster, "Value"=w305:i64)  [unwired: 2 in, 1 out]
        n184 = call "LCP Stop Pumping.vi"("error in (no error)"=w306, "Pump Handle"=w305) -> ()  [unwired: 9 in, 1 out]
        n185 = property on="Pump handle 2" class="DigNum (strict)"() -> (error out=w304:errorcluster, "Value"=w303:i64)  [unwired: 2 in, 1 out]
        n186 = call "LCP Stop Pumping.vi"("error in (no error)"=w304, "Pump Handle"=w303) -> ()  [unwired: 9 in, 1 out]
        n187 = property on="Pump handle 3" class="DigNum (strict)"() -> (error out=w311:errorcluster, "Value"=w310:i64)  [unwired: 2 in, 1 out]
        n188 = call "LCP Stop Pumping.vi"("error in (no error)"=w311, "Pump Handle"=w310) -> ()  [unwired: 9 in, 1 out]
      }
      event "SetSyringeLevel": Mouse Up {
        n189 = event-data() -> ()  [unwired: 1 in, 8 out]
        n190 = property on="Target Syr Level" class="DigNum (strict)"() -> ("Value"=w316:dbl)  [unwired: 2 in, 2 out]
        n191 = property on="Flow rate" class="DigNum (strict)"() -> ("Value"=w315:dbl)  [unwired: 2 in, 2 out]
        n192 = property on="Pump handle" class="DigNum (strict)"() -> ("Value"=w317:i64)  [unwired: 2 in, 2 out]
        n193 = call "LCP Set Fill Level.vi"("Flow"=w315, "Level"=w316, "Pump Handle"=w317) -> ()  [unwired: 8 in, 1 out]
      }
      event "SetSyringeLevel 2": Mouse Up {
        n194 = event-data() -> ()  [unwired: 1 in, 8 out]
        n195 = property on="Target Syr Level 2" class="DigNum (strict)"() -> ("Value"=w322:dbl)  [unwired: 2 in, 2 out]
        n196 = property on="Flow rate 2" class="DigNum (strict)"() -> ("Value"=w321:dbl)  [unwired: 2 in, 2 out]
        n197 = property on="Pump handle 2" class="DigNum (strict)"() -> ("Value"=w323:i64)  [unwired: 2 in, 2 out]
        n198 = call "LCP Set Fill Level.vi"("Flow"=w321, "Level"=w322, "Pump Handle"=w323) -> ()  [unwired: 8 in, 1 out]
      }
      event "SetSyringeLevel 3": Mouse Up {
        n199 = event-data() -> ()  [unwired: 1 in, 8 out]
        n200 = property on="Target Syr Level 3" class="DigNum (strict)"() -> ("Value"=w328:dbl)  [unwired: 2 in, 2 out]
        n201 = property on="Flow rate 3" class="DigNum (strict)"() -> ("Value"=w327:dbl)  [unwired: 2 in, 2 out]
        n202 = property on="Pump handle 3" class="DigNum (strict)"() -> ("Value"=w329:i64)  [unwired: 2 in, 2 out]
        n203 = call "LCP Set Fill Level.vi"("Flow"=w327, "Level"=w328, "Pump Handle"=w329) -> ()  [unwired: 8 in, 1 out]
      }
      event "Refill": Mouse Up {
        n204 = event-data() -> ()  [unwired: 1 in, 8 out]
        n205 = property on="Pump handle" class="DigNum (strict)"() -> (error out=w340:errorcluster, "Value"=w336:i64)  [unwired: 2 in, 1 out]
        n206 = call "LCP Get Volume Max.vi"("error in (no error)"=w340, "Pump Handle"=w336) -> ("error out"=w339:errorcluster, "Maximum Volume"=w337:dbl)  [unwired: 8 in]
        n207 = call "LCP Get Flow Rate Max.vi"("error in (no error)"=w339, "Pump Handle"=w336) -> ("error out"=w338:errorcluster, "Maximum Flow Rate"=w331:dbl)  [unwired: 8 in]
        n208 = Multiply(x=w331, y=0.3) -> (x*y=w330:dbl)
        n209 = call "LCP Set Fill Level.vi"("error in (no error)"=w338, "Flow"=w330, "Level"=w337, "Pump Handle"=w336) -> ()  [unwired: 7 in, 1 out]
      }
      event "Refill 2": Mouse Up {
        n210 = event-data() -> ()  [unwired: 1 in, 8 out]
        n211 = property on="Pump handle 2" class="DigNum (strict)"() -> (error out=w351:errorcluster, "Value"=w347:i64)  [unwired: 2 in, 1 out]
        n212 = call "LCP Get Volume Max.vi"("error in (no error)"=w351, "Pump Handle"=w347) -> ("error out"=w350:errorcluster, "Maximum Volume"=w348:dbl)  [unwired: 8 in]
        n213 = call "LCP Get Flow Rate Max.vi"("error in (no error)"=w350, "Pump Handle"=w347) -> ("error out"=w349:errorcluster, "Maximum Flow Rate"=w342:dbl)  [unwired: 8 in]
        n214 = Multiply(x=w342, y=0.3) -> (x*y=w341:dbl)
        n215 = call "LCP Set Fill Level.vi"("error in (no error)"=w349, "Flow"=w341, "Level"=w348, "Pump Handle"=w347) -> ()  [unwired: 7 in, 1 out]
      }
      event "Refill 3": Mouse Up {
        n216 = event-data() -> ()  [unwired: 1 in, 8 out]
        n217 = property on="Pump handle 3" class="DigNum (strict)"() -> (error out=w362:errorcluster, "Value"=w358:i64)  [unwired: 2 in, 1 out]
        n218 = call "LCP Get Volume Max.vi"("error in (no error)"=w362, "Pump Handle"=w358) -> ("error out"=w361:errorcluster, "Maximum Volume"=w359:dbl)  [unwired: 8 in]
        n219 = call "LCP Get Flow Rate Max.vi"("error in (no error)"=w361, "Pump Handle"=w358) -> ("error out"=w360:errorcluster, "Maximum Flow Rate"=w353:dbl)  [unwired: 8 in]
        n220 = Multiply(x=w353, y=0.3) -> (x*y=w352:dbl)
        n221 = call "LCP Set Fill Level.vi"("error in (no error)"=w360, "Flow"=w352, "Level"=w359, "Pump Handle"=w358) -> ()  [unwired: 7 in, 1 out]
      }
      event "Empty": Mouse Up {
        n222 = event-data() -> ()  [unwired: 1 in, 6 out]
        n223 = property on="Pump handle" class="DigNum (strict)"() -> ("Value"=w371:i64)  [unwired: 2 in, 2 out]
        n224 = call "LCP Get Flow Rate Max.vi"("Pump Handle"=w371) -> ("error out"=w370:errorcluster, "Maximum Flow Rate"=w364:dbl)  [unwired: 9 in]
        n225 = Multiply(x=w364, y=0.3) -> (x*y=w363:dbl)
        n226 = call "LCP Set Fill Level.vi"("error in (no error)"=w370, "Flow"=w363, "Level"=0.0, "Pump Handle"=w371) -> ()  [unwired: 7 in, 1 out]
      }
      event "Empty 2": Mouse Up {
        n227 = event-data() -> ()  [unwired: 1 in, 8 out]
        n228 = property on="Pump handle 2" class="DigNum (strict)"() -> ("Value"=w375:i64)  [unwired: 2 in, 2 out]
        n229 = call "LCP Get Flow Rate Max.vi"("Pump Handle"=w375) -> ("error out"=w380:errorcluster, "Maximum Flow Rate"=w373:dbl)  [unwired: 9 in]
        n230 = Multiply(x=w373, y=0.3) -> (x*y=w372:dbl)
        n231 = call "LCP Set Fill Level.vi"("error in (no error)"=w380, "Flow"=w372, "Level"=0.0, "Pump Handle"=w375) -> ()  [unwired: 7 in, 1 out]
      }
      event "Empty 3": Mouse Up {
        n232 = event-data() -> ()  [unwired: 1 in, 8 out]
        n233 = property on="Pump handle 3" class="DigNum (strict)"() -> ("Value"=w384:i64)  [unwired: 2 in, 2 out]
        n234 = call "LCP Get Flow Rate Max.vi"("Pump Handle"=w384) -> ("error out"=w389:errorcluster, "Maximum Flow Rate"=w382:dbl)  [unwired: 9 in]
        n235 = Multiply(x=w382, y=0.3) -> (x*y=w381:dbl)
        n236 = call "LCP Set Fill Level.vi"("error in (no error)"=w389, "Flow"=w381, "Level"=0.0, "Pump Handle"=w384) -> ()  [unwired: 7 in, 1 out]
      }
      event "Capture Path": Mouse Up {
        n237 = event-data() -> ()  [unwired: 1 in, 8 out]
        n238 = Path To String(path="Browse Capture Path") -> (string=w392:string)
        n239 = Current VI's Path() -> (path=w400:path)
        n240 = Build Path(base path=w400, name or relative path=path "../Py_tracker_2.py") -> (appended path=w398:path)
        n241 = node(w397, w398, "set_capture_path", w396, w392, "File Name") -> (w394:refnum<k35>, w393:errorcluster)  [unwired: 4 in, 2 out]
      }
    }
    "Communication Board" <- w22
    n242 = Or(x=w28, y=w30) -> (x .or. y?=w27:bool)
  }
  n243 = Bundle(FALSE, 0, "") -> (→"error out" →"error out 2" →"error out 3" →"Error out Python":errorcluster)  [unwired: 1 in]
  n244 = Close Python Session(session in=w16, error in=w17) -> ()  [unwired: 1 out]
  "Connected" <- FALSE ("Connected")
  "Syringe" <- 0.0
  "pumping" <- FALSE
  "Pump handle" <- i64 0 ("Pump handle")
  "Pump handle 2" <- i64 0 ("Pump handle")
  "Syringe 2" <- 0.0
  "Config Path" <- ""
  "pumping 2" <- FALSE
  "Syringe 3" <- 0.0
  "pumping 3" <- FALSE
  "Pump handle 3" <- i64 0 ("Pump handle")
